vi "Get Scalar Configuration.vi"(8 "error in (no error)":errorcluster, 9 "index":i32, 11 "Core Threads Configuration in":refnum<class "Core Threads Configuration.lvclass">) -> (0 "error out":errorcluster, 2 "thread configuration":T1={"processor"=-2, "priority offset"=0}, 3 "Core Threads Configuration out":refnum<class "Core Threads Configuration.lvclass">)   [LabVIEW 2017, in "DSF Core.lvlib" / "Core Threads Configuration.lvclass"]
uses:
  Core Threads Configuration.lvclass
  Configuration.ctl
  Core Threads Configuration.lvclass/Core Threads Configuration.ctl
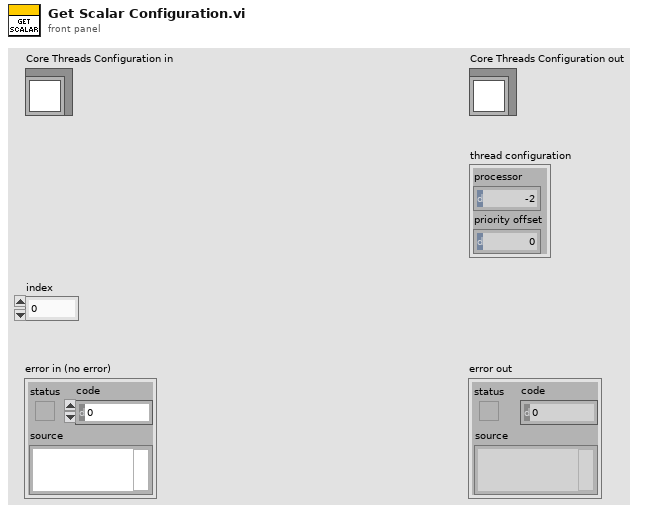
[diagram p1: front panel]
types:
  T1 = typedef "DSF Core.lvlib/Core Threads Configuration.lvclass/Configuration.ctl" = cluster{"processor":i32, "priority offset":i16}
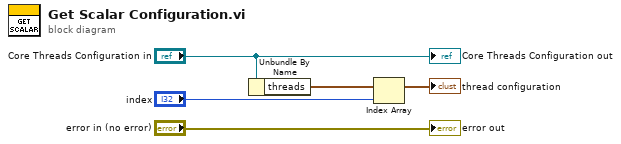
[diagram p0: block diagram]
diagram:
  n1 = Unbundle By Name("Core Threads Configuration in") -> ("threads"=w4:T1[])
  n2 = Index Array(array=w4, index="index") -> (element=→"thread configuration":T1)
  "error out" <- "error in (no error)"
  "Core Threads Configuration out" <- "Core Threads Configuration in"
